vi "Main.vi"(11 "Module Admin":refnum<class "Delacor_lib_QMH_Cloneable Module Admin.lvclass">) -> ()   [LabVIEW 2025, in "Power Supply.lvlib"]
doc: "This template is based off of the Queued Message Handler design pattern and the Queued Message Handler project template that ships with LabVIEW.\n\nThe main difference is that the queue is private to this module and communication between modules is performed via Broadcast and Request events.\n\nRequest events are wrapped in public API methods and are handled in the Event Handling Loop (EHL) of this VI. Any module can register for Broadcast events sent by this module. The EHL generates messages based on user interface actions.\n\nThe Message Handling Loop (MHL) processes messages generated by the EHL, or by other messages. The messages are string values, so new messages can be added easily to the Message Cases case structure in the MHL. Each message cluster can also provide an optional value for Message Data, which is a variant that can be converted to whatever message-specific data is required.\n_____\nBased on DQMH Dev Tools: Project Template 7.1.2.1547."
uses:
  Power Supply.lvlib
  <vilib>/Delacor/Delacor QMH/Libraries/Message Queue_class/Delacor_lib_QMH_Message Queue.lvclass/Delacor_lib_QMH_Message Queue.ctl
  <vilib>/Delacor/Delacor QMH/Libraries/Cloneable Module Admin_class/Delacor_lib_QMH_Cloneable Module Admin.lvclass/Delacor_lib_QMH_Cloneable Module Admin.ctl
  <vilib>/Delacor/Delacor QMH/Libraries/Module Admin_class/Delacor_lib_QMH_Module Admin.lvclass/Delacor_lib_QMH_Module Admin.ctl
  <vilib>/Delacor/Delacor QMH/Libraries/Message Queue_class/Delacor_lib_QMH_Message Queue.lvclass
  Module Data--cluster.ctl
  <vilib>/Utility/miscctls.llb/LVPointTypeDef.ctl
  <vilib>/Delacor/Delacor QMH/Libraries/Message Queue_class/Delacor_lib_QMH_Enqueue Message (Single).vi
  Stop Argument--cluster.ctl
  <vilib>/Delacor/Delacor QMH/Libraries/Cloneable Module Admin_class/Delacor_lib_QMH_Cloneable Module Admin.lvclass
  select child (Reply Payload)--cluster.ctl
  Classes/hardware-selection.ctl
  select child Argument--cluster.ctl
  Classes/generic-power-supply/generic-power-supply.lvclass
  Classes/PSP-603/PSP-603.lvclass
  read config (Reply Payload)--cluster.ctl
  read config Argument--cluster.ctl
  init device (Reply Payload)--cluster.ctl
  init device Argument--cluster.ctl
  close (Reply Payload)--cluster.ctl
  close Argument--cluster.ctl
  output (Reply Payload)--cluster.ctl
  output Argument--cluster.ctl
  set voltage (Reply Payload)--cluster.ctl
  set voltage Argument--cluster.ctl
  set current (Reply Payload)--cluster.ctl
  set current Argument--cluster.ctl
  C:/Users/grove/Desktop/LabVIEW/Git/dqmh-lvoop-template/Libraries/Power Supply/Classes/generic-power-supply/generic-power-supply.lvclass
  C:/Users/grove/Desktop/LabVIEW/Git/dqmh-lvoop-template/Libraries/Power Supply/Classes/PSP-603/PSP-603.lvclass
panel:
  out "error out":errorcluster
  out "Status":string
  in  "Simulate EHL Error":bool
  in  "Simulate MHL Error":bool
  # "Other processes communicate with this Module via its Public API (wrappers for its Request Events).\n\nThis Module communicates with other processes via its Broadcast Events.\nAny process that wants to receive these messages can register for this module's Broadcast events."
  # "This template is for the DQMH framework. See the block diagram for more information on how to use this template."
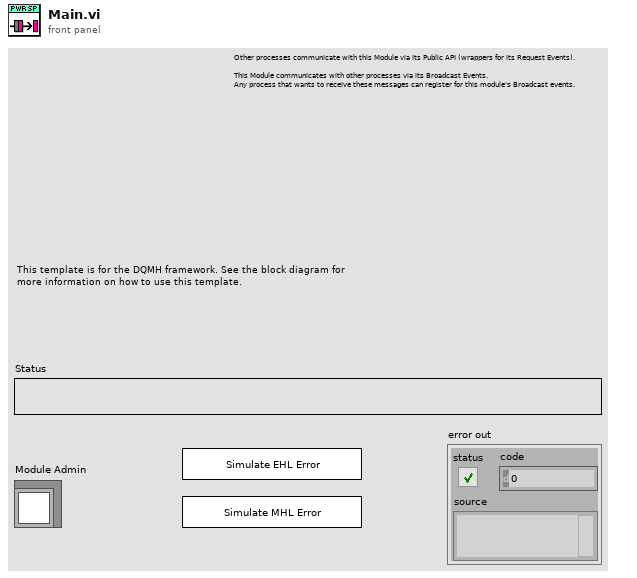
[diagram p1: front panel]
types:
  T1 = typedef "Power Supply.lvlib/Request Events--cluster.ctl" = cluster{"Stop Module":refnum<user-event>, "Show Panel":refnum<user-event>, "Hide Panel":refnum<user-event>, "Show Diagram":refnum<user-event>, "Get Module Execution Status":refnum<user-event>, "select child":refnum<user-event>, "read config":refnum<user-event>, "init device":refnum<user-event>, "close":refnum<user-event>, "output":refnum<user-event>, "set voltage":refnum<user-event>, "set current":refnum<user-event>}
  T2 = typedef "Power Supply.lvlib/Module Data--cluster.ctl" = cluster{"Status":string, "Power Supply Object":refnum<class "generic-power-supply.lvclass">}
  T3 = enum32{"invalid lock state", "Not Locked", "Locked (No Password)", "Password-protected"}
  T4 = typedef "Power Supply.lvlib/Stop Argument--cluster.ctl" = cluster{"Module ID":i32, "Origin":string, "Exit via Stop Module Req?":bool, "Wait for Module to stop?":bool}
  T5 = typedef "Power Supply.lvlib/select child Argument--cluster.ctl" = cluster{"Module ID":i32, "Enum":T6, "Wait Notifier":refnum<notifier>, "wait for reply":bool}
  T6 = typedef "hardware-selection.ctl" = enum16{"Parent", "Simulation", "PSP-603"}
  T7 = typedef "Power Supply.lvlib/read config Argument--cluster.ctl" = cluster{"Module ID":i32, "config json file":path, "Wait Notifier":refnum<notifier>, "wait for reply":bool}
  T8 = typedef "Power Supply.lvlib/init device Argument--cluster.ctl" = cluster{"Module ID":i32, "Variant":variant, "Wait Notifier":refnum<notifier>, "wait for reply":bool}
  T9 = typedef "Power Supply.lvlib/close Argument--cluster.ctl" = cluster{"Module ID":i32, "Wait Notifier":refnum<notifier>, "wait for reply":bool}
  T10 = typedef "Power Supply.lvlib/output Argument--cluster.ctl" = cluster{"Module ID":i32, "Output On/Off":bool, "Wait Notifier":refnum<notifier>, "wait for reply":bool}
  T11 = typedef "Power Supply.lvlib/set voltage Argument--cluster.ctl" = cluster{"Module ID":i32, "Output Voltage":dbl, "Wait Notifier":refnum<notifier>, "wait for reply":bool}
  T12 = typedef "Power Supply.lvlib/set current Argument--cluster.ctl" = cluster{"Module ID":i32, "Output Current":dbl, "Wait Notifier":refnum<notifier>, "wait for reply":bool}
  T13 = typedef "LVPointTypeDef.ctl" = cluster{"Horizontal":i16, "Vertical":i16}
  T14 = enum32{"Invalid", "Standard", "Closed", "Hidden", "Minimized", "Maximized"}
  T15 = typedef "Power Supply.lvlib/select child (Reply Payload)--cluster.ctl" = cluster{"Module ID":i32, "error":errorcluster}
  T16 = typedef "Power Supply.lvlib/read config (Reply Payload)--cluster.ctl" = cluster{"Module ID":i32, "error":errorcluster}
  T17 = typedef "Power Supply.lvlib/init device (Reply Payload)--cluster.ctl" = cluster{"Module ID":i32, "error":errorcluster}
  T18 = typedef "Power Supply.lvlib/close (Reply Payload)--cluster.ctl" = cluster{"Module ID":i32, "error":errorcluster}
  T19 = typedef "Power Supply.lvlib/output (Reply Payload)--cluster.ctl" = cluster{"Module ID":i32, "error":errorcluster}
  T20 = typedef "Power Supply.lvlib/set voltage (Reply Payload)--cluster.ctl" = cluster{"Module ID":i32, "error":errorcluster}
  T21 = typedef "Power Supply.lvlib/set current (Reply Payload)--cluster.ctl" = cluster{"Module ID":i32, "error":errorcluster}
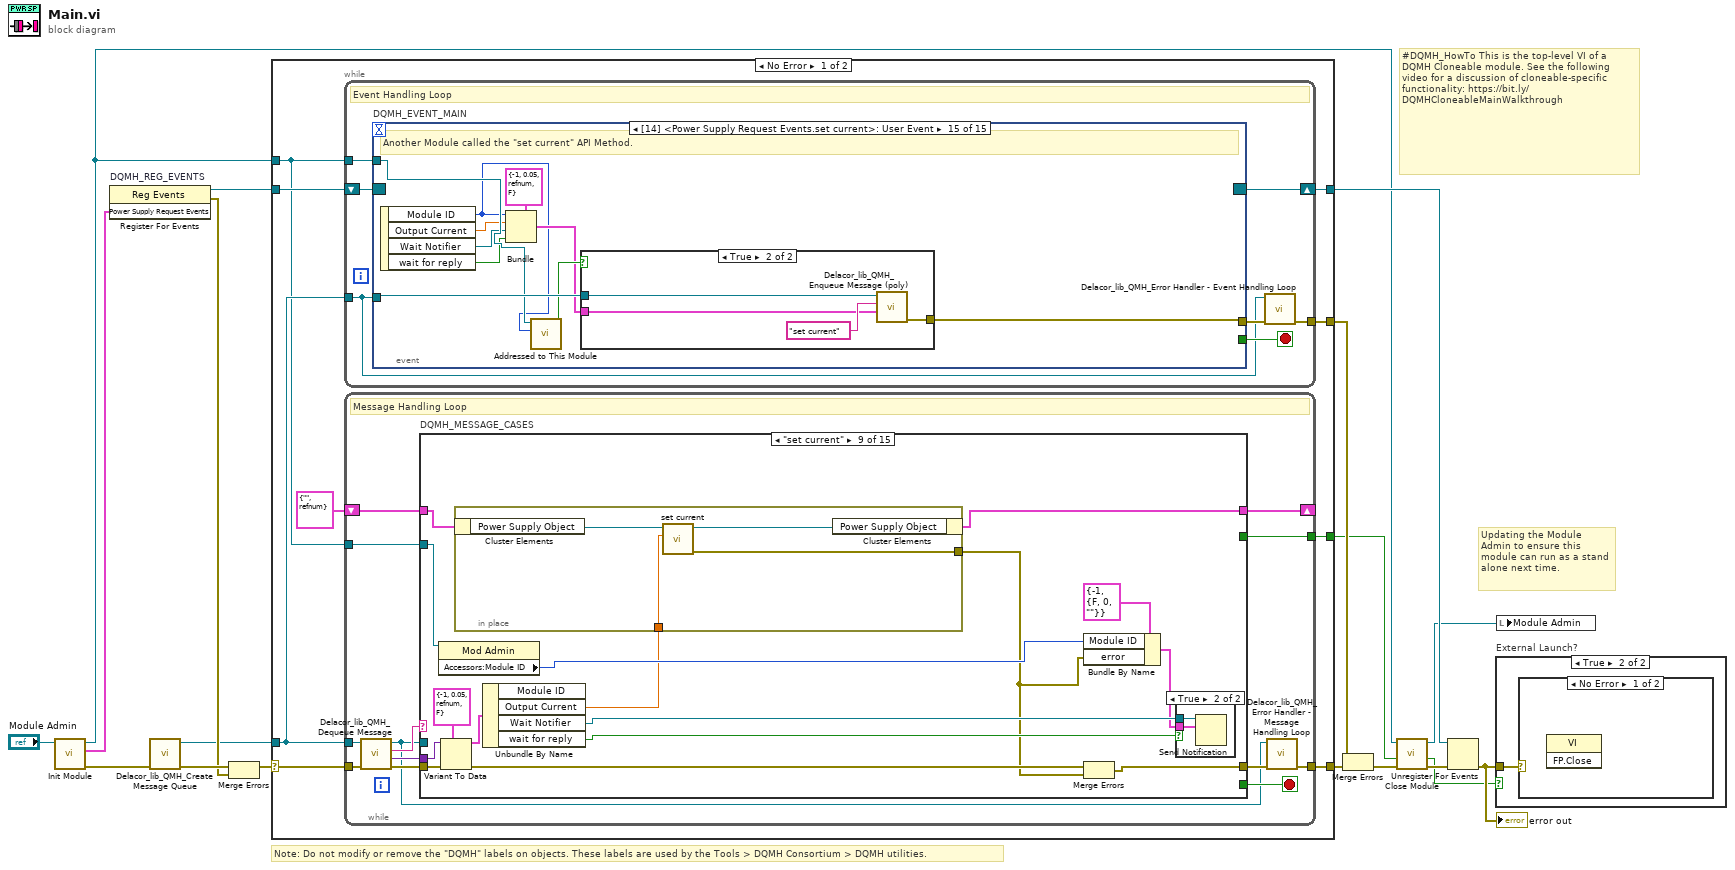
[diagram p0: block diagram]
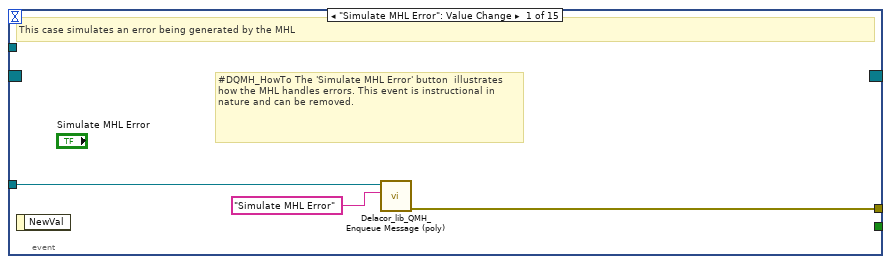
[diagram p2: hidden frame]
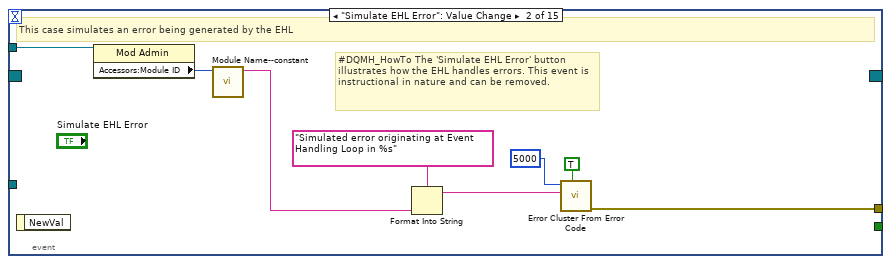
[diagram p3: hidden frame]
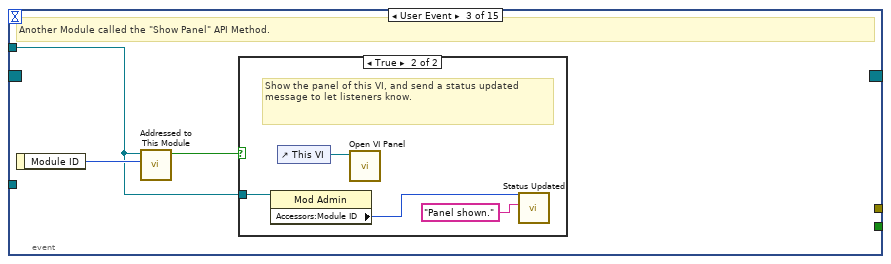
[diagram p4: hidden frame]
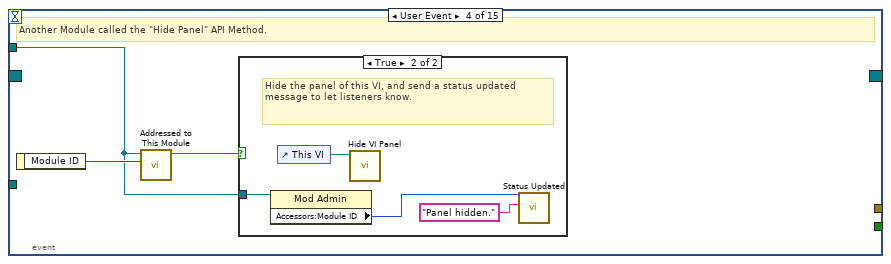
[diagram p6: hidden frame]
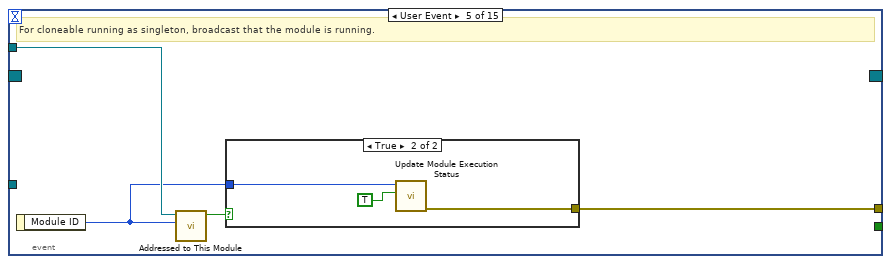
[diagram p8: hidden frame]
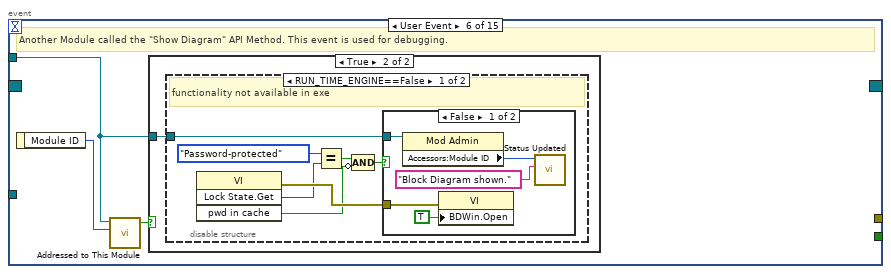
[diagram p10: hidden frame]
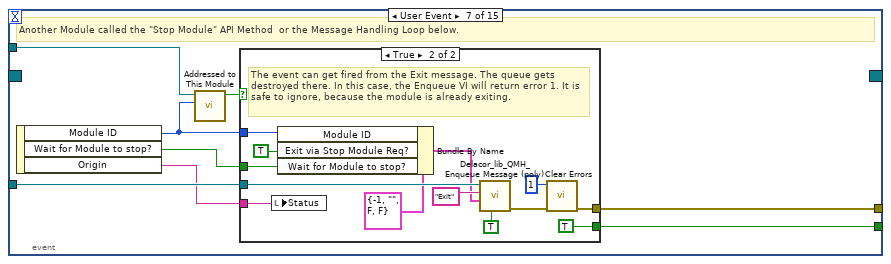
[diagram p14: hidden frame]
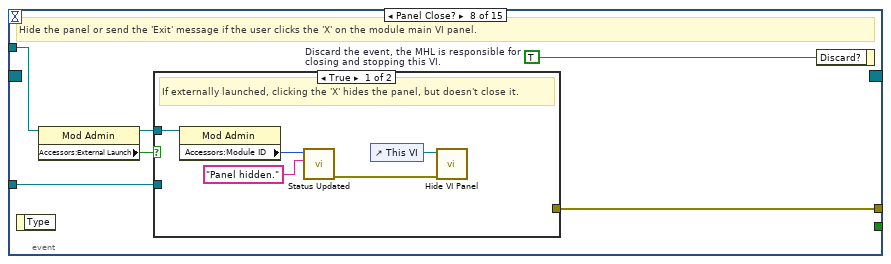
[diagram p16: hidden frame]
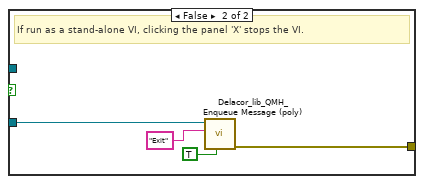
[diagram p17: hidden frame]
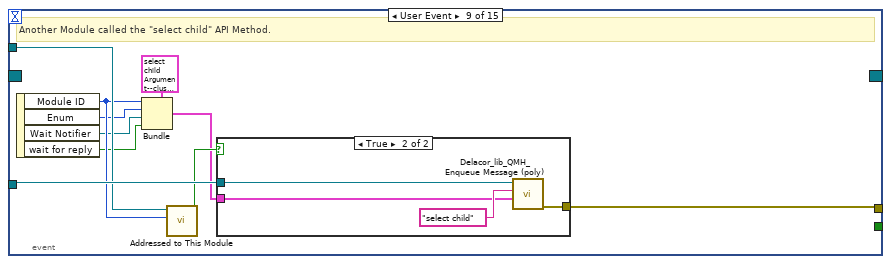
[diagram p18: hidden frame]
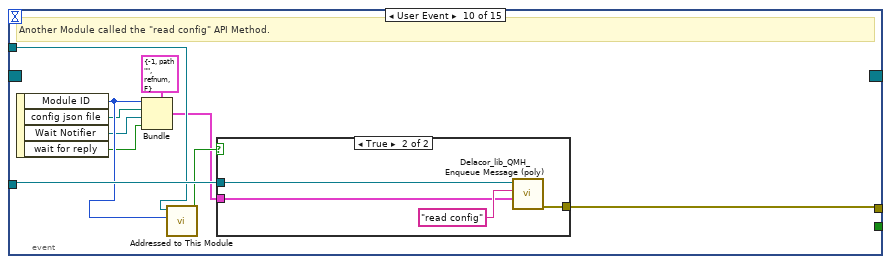
[diagram p20: hidden frame]
diagram:
  # "#DQMH_HowTo This is the top-level VI of a DQMH Cloneable module. See the following video for a discussion of cloneable-specific functionality: https://bit.ly/DQMHCloneableMainWalkthrough"
  # "Note: Do not modify or remove the \"DQMH\" labels on objects. These labels are used by the Tools > DQMH Consortium > DQMH utilities."
  # "Updating the Module Admin to ensure this module can run as a stand alone next time."
  n1 = call "Init Module.vi"("Cloneable Module Admin in"="Module Admin") -> ("error out"=w15:errorcluster, "Power Supply Request Events"=w7:T1, "Cloneable Module Admin out"=w4:refnum<class "Delacor_lib_QMH_Cloneable Module Admin.lvclass">)  [unwired: 8 in]
  n2 = register-events "DQMH_REG_EVENTS"(w7) -> (reference out=w8:refnum<event-registration>, error out=w10:errorcluster)  [unwired: 2 in]
  n3 = call <vilib>:"Delacor_lib_QMH_Create Message Queue.vi"("error in"=w15) -> ("error out"=w12:errorcluster, "Message Queue"=w6:refnum<class "Delacor_lib_QMH_Message Queue.lvclass">)  [unwired: 9 in]
  n4 = Merge Errors(w12, w10) -> (w11:errorcluster)
  n5 = case shown="No Error" w11 {
    selector: w11 -> [w25 w477]
    tunnel: [w27 w476] -> w16
    tunnel: [w24 w475] -> w9
    tunnel: w8 -> [w22 w475]
    tunnel: w6 -> [w21 w468]
    tunnel: [w26 _] -> w17
    tunnel: w4 -> [w20 w471]
    tunnel: [w19 _] -> w2
    frame No Error {
      n6 = while {
        tunnel: w21 -> [w28]
        shift-right: [w31] -> w24
        shift-left: w22 -> [w32]
        tunnel: [w33] -> w26
        tunnel: w20 -> [w29]
        stop <- w30 stop-if-true
        # "Event Handling Loop"
        n7 = event "DQMH_EVENT_MAIN" shown="[14] <Power Supply Request Events.set current>: User Event" {
          selector: w32 -> [_ _ _ _ _ _ _ _ _ _ _ _ _ _ _]
          dyn-events: [_ _ _ _ _ _ _ _ _ _ _ _ _ _ _] -> w31
          timeout: _ -> [_ _ _ _ _ _ _ _ _ _ _ _ _ _ _]
          tunnel: [_ _ _ _ _ _ w86 _ _ _ _ _ _ _ _] -> w30
          tunnel: w28 -> [w36 _ _ _ _ _ w89 w106 w128 w142 w156 w169 w183 w197 w211]
          tunnel: [w37 w45 _ _ w63 _ w90 w109 w119 w133 w147 w161 w174 w188 w202] -> w34
          tunnel: w29 -> [_ w44 w46 w53 w61 w67 w88 w107 w126 w140 w154 w167 w181 w195 w209]
          event "Simulate MHL Error": Value Change {
            # "#DQMH_HowTo The 'Simulate MHL Error' button  illustrates how the MHL handles errors. This event is instructional in nature and can be removed."
            # "This case simulates an error being generated by the MHL"
            n8 = event-data() -> ()  [unwired: 1 in, 1 out]
            n9 = call-poly <vilib>:"Delacor_lib_QMH_Enqueue Message (poly).vi"("Message"="Simulate MHL Error", "Message Queue in"=w36) -> ("error out"=w37:errorcluster)  [unwired: 8 in, 1 out]
          }
          event "Simulate EHL Error": Value Change {
            # "#DQMH_HowTo The 'Simulate EHL Error' button  illustrates how the EHL handles errors. This event is instructional in nature and can be removed."
            # "This case simulates an error being generated by the EHL"
            n10 = event-data() -> ()  [unwired: 1 in, 1 out]
            n11 = property on="Property Node" class="Mod Admin"(reference=w44) -> ("Accessors:Module ID"=w43:i32)  [unwired: 1 in, 2 out]
            n12 = call "Module Name--constant.vi"("Module ID"=w43) -> ("Module Name"=w38:string)  [unwired: 10 in]
            n13 = Format Into String(format string="Simulated error originating at Event Handling Loop in %s", w38) -> (resulting string=w41:string)  [unwired: 2 in, 1 out]
            n14 = call <vilib>:"Error Cluster From Error Code.vi"("show call chain? (False)"=TRUE, "error message (\"\")"=w41, "error code (0)"=5000) -> ("error out"=w45:errorcluster)  [unwired: 6 in]
          }
          event User Event {
            # "Another Module called the \"Show Panel\" API Method."
            n15 = event-data() -> ("Module ID"=w47:i32)  [unwired: 1 in]
            n16 = call "Addressed to This Module.vi"("Module ID from Argument"=w47, "Module Admin"=w46) -> ("Addressed to this instance?"=w48:bool)  [unwired: 8 in, 1 out]
            n17 = case shown="True" w48 {
              tunnel: w46 -> [_ w50]
              frame False {
              }
              frame True {
                # "Show the panel of this VI, and send a status updated message to let listeners know."
                n18 = property on="Property Node" class="Mod Admin"(reference=w50) -> ("Accessors:Module ID"=w49:i32)  [unwired: 1 in, 2 out]
                n19 = control-ref of="This VI"() -> (w52:refnum<vi>)
                n20 = call "Open VI Panel.vi"("VI"=w52) -> ()  [unwired: 10 in, 1 out]
                n21 = call "Status Updated.vi"("Status"="Panel shown." ("format string"), "Module ID"=w49) -> ()  [unwired: 9 in, 1 out]
              }
            }
          }
          event User Event {
            # "Another Module called the \"Hide Panel\" API Method."
            n22 = event-data() -> ("Module ID"=w54:i32)  [unwired: 1 in]
            n23 = call "Addressed to This Module.vi"("Module ID from Argument"=w54, "Module Admin"=w53) -> ("Addressed to this instance?"=w55:bool)  [unwired: 8 in, 1 out]
            n24 = case shown="True" w55 {
              tunnel: w53 -> [_ w57]
              frame False {
              }
              frame True {
                # "Hide the panel of this VI, and send a status updated message to let listeners know."
                n25 = property on="Property Node" class="Mod Admin"(reference=w57) -> ("Accessors:Module ID"=w56:i32)  [unwired: 1 in, 2 out]
                n26 = control-ref of="This VI"() -> (w59:refnum<vi>)
                n27 = call "Hide VI Panel.vi"("VI"=w59) -> ()  [unwired: 10 in, 1 out]
                n28 = call "Status Updated.vi"("Status"="Panel hidden." ("format string"), "Module ID"=w56) -> ()  [unwired: 9 in, 1 out]
              }
            }
          }
          event User Event {
            # "For cloneable running as singleton, broadcast that the module is running."
            n29 = event-data() -> ("Module ID"=w60:i32)  [unwired: 1 in]
            n30 = call "Addressed to This Module.vi"("Module ID from Argument"=w60, "Module Admin"=w61) -> ("Addressed to this instance?"=w62:bool)  [unwired: 8 in, 1 out]
            n31 = case shown="True" w62 {
              tunnel: [_ w66] -> w63
              tunnel: w60 -> [_ w65]
              frame False {
              }
              frame True {
                n32 = call "Update Module Execution Status.vi"("Running?"=TRUE, "Module ID"=w65) -> ("error out"=w66:errorcluster)  [unwired: 9 in]
              }
            }
          }
          event User Event {
            # "Another Module called the \"Show Diagram\" API Method. This event is used for debugging."
            n33 = event-data() -> ("Module ID"=w68:i32)  [unwired: 1 in]
            n34 = call "Addressed to This Module.vi"("Module ID from Argument"=w68, "Module Admin"=w67) -> ("Addressed to this instance?"=w69:bool)  [unwired: 8 in, 1 out]
            n35 = case shown="True" w69 {
              tunnel: w67 -> [_ w70]
              frame False {
              }
              frame True {
                n36 = disable-structure shown="RUN_TIME_ENGINE==False" {
                  disable-tunnel: w70 -> [w71 _]
                  frame condition #0 (active) {
                    # "functionality not available in exe"
                    n37 = invoke on="Invoke Node" class="VI" method="Lock State.Get"() -> (error out=w77:errorcluster, "Get Lock State"=w76:T3, "pwd in cache"=w73:bool)  [unwired: 4 in, 1 out]
                    n38 = Equal?(x=T3."Password-protected", y=w76) -> (x = y?=w74:bool)
                    n39 = Compound Arithmetic op=AND(w74, invert w73) -> (w72:bool)
                    n40 = case shown="False" w72 {
                      tunnel: w77 -> [w82 _]
                      tunnel: w71 -> [w79 _]
                      frame False {
                        n41 = property on="Property Node" class="Mod Admin"(reference=w79) -> ("Accessors:Module ID"=w78:i32)  [unwired: 1 in, 2 out]
                        n42 = property on="Property Node" class="VI"(error in=w82, "BDWin.Open"=TRUE ("Block Diagram Window:Open")) -> ()  [unwired: 1 in, 2 out]
                        n43 = call "Status Updated.vi"("Status"="Block Diagram shown." ("format string"), "Module ID"=w78) -> ()  [unwired: 9 in, 1 out]
                      }
                      frame True {
                        # "Password-protected VI, and the password is not in the cache. Do not show the diagram."
                      }
                    }
                  }
                  frame condition #1 {
                  }
                }
              }
            }
          }
          event User Event {
            # "Another Module called the \"Stop Module\" API Method  or the Message Handling Loop below."
            n44 = event-data() -> ("Module ID"=w84:i32, "Wait for Module to stop?"=w85:bool, "Origin"=w83:string)  [unwired: 1 in]
            n45 = call "Addressed to This Module.vi"("Module ID from Argument"=w84, "Module Admin"=w88) -> ("Addressed to this instance?"=w87:bool)  [unwired: 8 in, 1 out]
            n46 = case shown="True" w87 {
              tunnel: [_ w102] -> w90
              tunnel: w89 -> [_ w98]
              tunnel: [_ TRUE] -> w86
              tunnel: w85 -> [_ w93]
              tunnel: w84 -> [_ w95]
              tunnel: w83 -> [_ w91]
              frame False {
              }
              frame True {
                # "The event can get fired from the Exit message. The queue gets destroyed there. In this case, the Enqueue VI will return error 1. It is safe to ignore, because the module is already exiting."
                n47 = local write "Status"(w91) -> ()
                n48 = Bundle By Name(cluster=T4 {"Module ID"=-1, "Origin"="", "Exit via Stop Module Req?"=FALSE, "Wait for Module to stop?"=FALSE} ("Stop Argument"), "Module ID"=w95, "Exit via Stop Module Req?"=TRUE, "Wait for Module to stop?"=w93) -> (w92:T4)
                n49 = call-poly <vilib>:"Delacor_lib_QMH_Enqueue Message (poly).vi"("Priority Message? (F)"=TRUE, "Message Data"=w92, "Message"="Exit", "Message Queue in"=w98) -> ("error out"=w103:errorcluster)  [unwired: 6 in, 1 out]
                n50 = call <vilib>:"Clear Errors.vi"("error in (no error)"=w103, "specific error code to clear (0: all)"=1) -> ("error out"=w102:errorcluster)  [unwired: 4 in, 1 out]
              }
            }
          }
          event Panel Close? {
            w108 = TRUE  # Discard the event, the MHL is responsible for closing and stopping this VI.
            # "Hide the panel or send the 'Exit' message if the user clicks the 'X' on the module main VI panel."
            n51 = event-data() -> ()  [unwired: 1 in, 1 out]
            n52 = property on="Property Node" class="Mod Admin"(reference=w107) -> (reference out=w104:refnum<class "Delacor_lib_QMH_Cloneable Module Admin.lvclass">, "Accessors:External Launch"=w105:bool)  [unwired: 1 in, 1 out]
            n53 = case shown="True" w105 {
              tunnel: w106 -> [_ w117]
              tunnel: [_ w118] -> w109
              tunnel: w104 -> [w112 _]
              frame True {
                # "If externally launched, clicking the 'X' hides the panel, but doesn't close it."
                n54 = property on="Property Node" class="Mod Admin"(reference=w112) -> ("Accessors:Module ID"=w111:i32)  [unwired: 1 in, 2 out]
                n55 = call "Status Updated.vi"("Status"="Panel hidden." ("format string"), "Module ID"=w111) -> ("error out"=w110:errorcluster)  [unwired: 9 in]
                n56 = control-ref of="This VI"() -> (w114:refnum<vi>)
                n57 = call "Hide VI Panel.vi"("error in"=w110, "VI"=w114) -> ()  [unwired: 9 in, 1 out]
              }
              frame False {
                # "If run as a stand-alone VI, clicking the panel 'X' stops the VI."
                n58 = call-poly <vilib>:"Delacor_lib_QMH_Enqueue Message (poly).vi"("Priority Message? (F)"=TRUE, "Message"="Exit", "Message Queue in"=w117) -> ("error out"=w118:errorcluster)  [unwired: 7 in, 1 out]
              }
            }
            n59 = event-data ("Event Filter Node")("Discard?"=w108) -> ()  [unwired: 1 in, 1 out]
          }
          event User Event {
            # "Another Module called the \"select child\" API Method."
            n60 = event-data() -> ("Module ID"=w123:i32, "Enum"=w122:T6, "Wait Notifier"=w121:refnum<notifier>, "wait for reply"=w120:bool)  [unwired: 1 in]
            n61 = Bundle(cluster=T5 {"Module ID"=-1, "Enum"=enum."PSP-603", "Wait Notifier"=refnum, "wait for reply"=FALSE} ("select child Argument"), "Module ID"=w123, "Enum"=w122, "Wait Notifier"=w121, "wait for reply"=w120) -> (w124:T5)
            n62 = call "Addressed to This Module.vi"("Module ID from Argument"=w123, "Module Admin"=w126) -> ("Addressed to this instance?"=w127:bool)  [unwired: 8 in, 1 out]
            n63 = case shown="True" w127 {
              tunnel: w128 -> [_ w132]
              tunnel: w124 -> [_ w130]
              tunnel: [_ w129] -> w119
              frame False {
              }
              frame True {
                n64 = call-poly <vilib>:"Delacor_lib_QMH_Enqueue Message (poly).vi"("Message Data"=w130, "Message"="select child", "Message Queue in"=w132) -> ("error out"=w129:errorcluster)  [unwired: 7 in, 1 out]
              }
            }
          }
          event User Event {
            # "Another Module called the \"read config\" API Method."
            n65 = event-data() -> ("Module ID"=w137:i32, "config json file"=w136:path, "Wait Notifier"=w135:refnum<notifier>, "wait for reply"=w134:bool)  [unwired: 1 in]
            n66 = Bundle(cluster=T7 {"Module ID"=-1, "config json file"=path "", "Wait Notifier"=refnum, "wait for reply"=FALSE} ("read config Argument"), "Module ID"=w137, "config json file"=w136, "Wait Notifier"=w135, "wait for reply"=w134) -> (w138:T7)
            n67 = call "Addressed to This Module.vi"("Module ID from Argument"=w137, "Module Admin"=w140) -> ("Addressed to this instance?"=w141:bool)  [unwired: 8 in, 1 out]
            n68 = case shown="True" w141 {
              tunnel: w142 -> [_ w146]
              tunnel: w138 -> [_ w144]
              tunnel: [_ w143] -> w133
              frame False {
              }
              frame True {
                n69 = call-poly <vilib>:"Delacor_lib_QMH_Enqueue Message (poly).vi"("Message Data"=w144, "Message"="read config", "Message Queue in"=w146) -> ("error out"=w143:errorcluster)  [unwired: 7 in, 1 out]
              }
            }
          }
          event User Event {
            # "Another Module called the \"init device\" API Method."
            n70 = event-data() -> ("Module ID"=w151:i32, "Variant"=w150:variant, "Wait Notifier"=w149:refnum<notifier>, "wait for reply"=w148:bool)  [unwired: 1 in]
            n71 = Bundle(cluster=T8 {"Module ID"=-1, "Variant"=variant, "Wait Notifier"=refnum, "wait for reply"=FALSE} ("init device Argument"), "Module ID"=w151, "Variant"=w150, "Wait Notifier"=w149, "wait for reply"=w148) -> (w152:T8)
            n72 = call "Addressed to This Module.vi"("Module ID from Argument"=w151, "Module Admin"=w154) -> ("Addressed to this instance?"=w155:bool)  [unwired: 8 in, 1 out]
            n73 = case shown="True" w155 {
              tunnel: w156 -> [_ w160]
              tunnel: w152 -> [_ w158]
              tunnel: [_ w157] -> w147
              frame False {
              }
              frame True {
                n74 = call-poly <vilib>:"Delacor_lib_QMH_Enqueue Message (poly).vi"("Message Data"=w158, "Message"="init device", "Message Queue in"=w160) -> ("error out"=w157:errorcluster)  [unwired: 7 in, 1 out]
              }
            }
          }
          event User Event {
            # "Another Module called the \"close\" API Method."
            n75 = event-data() -> ("Module ID"=w164:i32, "Wait Notifier"=w163:refnum<notifier>, "wait for reply"=w162:bool)  [unwired: 1 in]
            n76 = Bundle(cluster=T9 {"Module ID"=-1, "Wait Notifier"=refnum, "wait for reply"=FALSE} ("close Argument"), "Module ID"=w164, "Wait Notifier"=w163, "wait for reply"=w162) -> (w165:T9)
            n77 = call "Addressed to This Module.vi"("Module ID from Argument"=w164, "Module Admin"=w167) -> ("Addressed to this instance?"=w168:bool)  [unwired: 8 in, 1 out]
            n78 = case shown="True" w168 {
              tunnel: w169 -> [_ w173]
              tunnel: w165 -> [_ w171]
              tunnel: [_ w170] -> w161
              frame False {
              }
              frame True {
                n79 = call-poly <vilib>:"Delacor_lib_QMH_Enqueue Message (poly).vi"("Message Data"=w171, "Message"="close", "Message Queue in"=w173) -> ("error out"=w170:errorcluster)  [unwired: 7 in, 1 out]
              }
            }
          }
          event User Event {
            # "Another Module called the \"output\" API Method."
            n80 = event-data() -> ("Module ID"=w178:i32, "Output On/Off"=w177:bool, "Wait Notifier"=w176:refnum<notifier>, "wait for reply"=w175:bool)  [unwired: 1 in]
            n81 = Bundle(cluster=T10 {"Module ID"=-1, "Output On/Off"=FALSE, "Wait Notifier"=refnum, "wait for reply"=FALSE} ("output Argument"), "Module ID"=w178, "Output On/Off"=w177, "Wait Notifier"=w176, "wait for reply"=w175) -> (w179:T10)
            n82 = call "Addressed to This Module.vi"("Module ID from Argument"=w178, "Module Admin"=w181) -> ("Addressed to this instance?"=w182:bool)  [unwired: 8 in, 1 out]
            n83 = case shown="True" w182 {
              tunnel: w183 -> [_ w187]
              tunnel: w179 -> [_ w185]
              tunnel: [_ w184] -> w174
              frame False {
              }
              frame True {
                n84 = call-poly <vilib>:"Delacor_lib_QMH_Enqueue Message (poly).vi"("Message Data"=w185, "Message"="output", "Message Queue in"=w187) -> ("error out"=w184:errorcluster)  [unwired: 7 in, 1 out]
              }
            }
          }
          event User Event {
            # "Another Module called the \"set voltage\" API Method."
            n85 = event-data() -> ("Module ID"=w192:i32, "Output Voltage"=w191:dbl, "Wait Notifier"=w190:refnum<notifier>, "wait for reply"=w189:bool)  [unwired: 1 in]
            n86 = Bundle(cluster=T11 {"Module ID"=-1, "Output Voltage"=10.0, "Wait Notifier"=refnum, "wait for reply"=FALSE} ("set voltage Argument"), "Module ID"=w192, "Output Voltage"=w191, "Wait Notifier"=w190, "wait for reply"=w189) -> (w193:T11)
            n87 = call "Addressed to This Module.vi"("Module ID from Argument"=w192, "Module Admin"=w195) -> ("Addressed to this instance?"=w196:bool)  [unwired: 8 in, 1 out]
            n88 = case shown="True" w196 {
              tunnel: w197 -> [_ w201]
              tunnel: w193 -> [_ w199]
              tunnel: [_ w198] -> w188
              frame False {
              }
              frame True {
                n89 = call-poly <vilib>:"Delacor_lib_QMH_Enqueue Message (poly).vi"("Message Data"=w199, "Message"="set voltage", "Message Queue in"=w201) -> ("error out"=w198:errorcluster)  [unwired: 7 in, 1 out]
              }
            }
          }
          event User Event {
            # "Another Module called the \"set current\" API Method."
            n90 = event-data() -> ("Module ID"=w206:i32, "Output Current"=w205:dbl, "Wait Notifier"=w204:refnum<notifier>, "wait for reply"=w203:bool)  [unwired: 1 in]
            n91 = Bundle(cluster=T12 {"Module ID"=-1, "Output Current"=0.05, "Wait Notifier"=refnum, "wait for reply"=FALSE} ("set current Argument"), "Module ID"=w206, "Output Current"=w205, "Wait Notifier"=w204, "wait for reply"=w203) -> (w207:T12)
            n92 = call "Addressed to This Module.vi"("Module ID from Argument"=w206, "Module Admin"=w209) -> ("Addressed to this instance?"=w210:bool)  [unwired: 8 in, 1 out]
            n93 = case shown="True" w210 {
              tunnel: w211 -> [_ w215]
              tunnel: w207 -> [_ w213]
              tunnel: [_ w212] -> w202
              frame False {
              }
              frame True {
                n94 = call-poly <vilib>:"Delacor_lib_QMH_Enqueue Message (poly).vi"("Message Data"=w213, "Message"="set current", "Message Queue in"=w215) -> ("error out"=w212:errorcluster)  [unwired: 7 in, 1 out]
              }
            }
          }
        }
        n95 = call-dynamic "Delacor_lib_QMH_Error Handler - Event Handling Loop.vi"("error in"=w34, "Message Queue in"=w28) -> ("dup error in"=w33:errorcluster)  [unwired: 8 in, 1 out]
      }
      n96 = while {
        tunnel: w21 -> [w216]
        shift-right: [w223] -> _
        shift-left: T2 {"Status"="", "Power Supply Object"=refnum} ("Data Cluster") -> [w224]
        tunnel: w25 -> [w227]
        tunnel: [w225] -> w27
        tunnel: w20 -> [w218]
        tunnel: [w217] -> w19
        stop <- w222 stop-if-true
        # "Message Handling Loop"
        n97 = call-dynamic "Delacor_lib_QMH_Dequeue Message.vi"("error in"=w227, "Message Queue in"=w216) -> ("error out"=w226:errorcluster, "Message Data"=w220:variant, "Message"=w221:string, "Message Queue out"=w219:refnum<class "Delacor_lib_QMH_Message Queue.lvclass">)  [unwired: 6 in]
        n98 = case "DQMH_MESSAGE_CASES" shown="\"set current\"" w221 {
          selector: w221 -> [_ _ _ _ _ _ _ _ _ _ _ _ _ _ w457]
          tunnel: w219 -> [_ _ _ _ _ _ _ _ _ _ _ w412 _ w449 _]
          tunnel: w226 -> [w247 w251 w267 w290 w312 w333 w354 w376 w398 w407 w409 w421 w438 w455 w466]
          tunnel: [w245 w251 w258 w281 w303 w324 w345 w367 w389 w406 w409 w417 w437 w450 w467] -> w228
          tunnel: w224 -> [w238 w250 w255 w278 w300 w321 w342 w364 w386 w405 w408 w416 w435 w448 w464]
          tunnel: [w237 w250 w254 w277 w299 w320 w341 w363 w385 w405 w408 w416 w435 w448 w464] -> w223
          tunnel: [_ _ _ _ _ _ _ _ _ _ _ _ _ w447 _] -> w222
          tunnel: w220 -> [_ _ w265 w288 w310 w331 w352 w374 w396 _ _ w415 _ w445 _]
          tunnel: w218 -> [w233 _ w256 w279 w301 w322 w343 w365 w387 _ _ w414 w433 w440 w463]
          tunnel: [_ _ _ _ _ _ _ _ _ _ _ _ _ w443 _] -> w217
          frame "Initialize" {
            w230 = "Initial Message" ("Initial Message")
            # "#DQMH_CodeNeeded - Initialize the appearance of the front panel."
            # "#DQMH_CodeNeeded - Initialize your state data here."
            # "Initialize - Any operation that needs to be done before the module can receive messages. Synchronize Caller Events.vi will inform Start Module.vi that the module has launched and is ready to receive messages. Module Did Init.vi will broadcast that the module initialized."
            n99 = call "Synchronize Caller Events.vi"("error in"=w247, "Module Admin"=w233) -> ("error out"=w246:errorcluster, "Module Admin out"=w232:refnum<class "Delacor_lib_QMH_Cloneable Module Admin.lvclass">)  [unwired: 8 in]
            n100 = property on="Property Node" class="Mod Admin"(reference=w232) -> ("Accessors:Module ID"=w229:i32, "Accessors:External Launch"=w234:bool)  [unwired: 1 in, 2 out]
            n101 = call "Module Name--constant.vi"("Module ID"=w229) -> ("Module Name"=w242:string)  [unwired: 10 in]
            n102 = property on="Property Node" class="VI"("Front Panel.Title"=w242) -> (reference out=w244:refnum<vi>, error out=w249:errorcluster)  [unwired: 2 in]
            n103 = Select(t=T14."Hidden" ("State"), s=w234, f=T14."Standard" ("State")) -> (s? t:f=w239:T14)
            n104 = invoke on="Invoke Node" class="VI" method="FP.Open"(reference=w244, error in=w249, "State"=w239) -> (reference out=w243:refnum<vi>, error out=w248:errorcluster)  [unwired: 2 in, 3 out]
            n105 = Bundle By Name(cluster=w238, "Status"=w230) -> (w237:T2)
            n106 = invoke on="Invoke Node" class="VI" method="FP.Center"(reference=w243, error in=w248) -> ()  [unwired: 1 in, 3 out]
            n107 = property on="Pane" class="Pane"("Origin"=T13 {"Horizontal"=0, "Vertical"=0}) -> ()  [unwired: 2 in, 2 out]
            n108 = call "Module Name--constant.vi"("Module ID"=w229) -> ("Module Name"=w235:string)  [unwired: 10 in]
            n109 = call "Module Did Init.vi"("error in"=w246, "Initialized?"=TRUE, "Origin"=w235, "Module ID"=w229) -> ("error out"=w245:errorcluster)  [unwired: 7 in]
            "Status" <- w230
          }
          frame "---Module Specific---" {
            # "Separator -- The following cases handle messages specific to this Module."
          }
          frame "select child" {
            w253 = errorcluster {"status"=FALSE, "code"=0, "source"=""} ("error")
            n110 = Variant To Data(error in=w267, type=T5 {"Module ID"=-1, "Enum"=enum."PSP-603", "Wait Notifier"=refnum, "wait for reply"=FALSE} ("select child Argument"), Variant=w265) -> (data=w263:T5, error out=w266:errorcluster)
            n111 = property class="Mod Admin"(reference=w256) -> ("Accessors:Module ID"=w257:i32)  [unwired: 1 in, 2 out]
            n112 = Unbundle By Name(w263) -> ("Enum"=w252:T6, "Wait Notifier"=w262:refnum<notifier>, "wait for reply"=w261:bool)  [unwired: 1 out]
            n113 = in-place {
              in-place-border: w252 -> [w268]
              n114 = in-place-cluster #1(w255) -> ()  [unwired: 1 out]
              n115 = case shown="\"Parent\"" w268 {
                tunnel: [refnum<class "generic-power-supply.lvclass"> refnum ("Power Supply.lvlib:generic-power-supply.lvclass") refnum<class "generic-power-supply.lvclass"> refnum ("Power Supply.lvlib:generic-power-supply.lvclass") refnum<class "PSP-603.lvclass"> refnum ("Power Supply.lvlib:PSP-603.lvclass")] -> w269
                frame "Simulation" {
                }
                frame "Parent" {
                }
                frame "PSP-603" {
                }
              }
              n116 = in-place-cluster #1("Power Supply Object"=w269) -> (w254:T2)
            }
            n117 = Bundle By Name(cluster=T15 {"Module ID"=-1, "error"={"status"=FALSE, "code"=0, "source"=""}} ("select child (Reply Payload)"), "Module ID"=w257, "error"=w253) -> (w260:T15)
            n118 = Merge Errors(w266, w253) -> (w258:errorcluster)
            n119 = case "DQMH_FIRE_NOTIFIER" shown="True" w261 {
              tunnel: w262 -> [_ w274]
              tunnel: w260 -> [_ w273]
              frame False {
              }
              frame True {
                n120 = Send Notification(notification=w273, notifier=w274) -> ()  [unwired: 1 in, 2 out]
              }
            }
          }
          frame "read config" {
            n121 = Variant To Data(error in=w290, type=T7 {"Module ID"=-1, "config json file"=path "", "Wait Notifier"=refnum, "wait for reply"=FALSE} ("read config Argument"), Variant=w288) -> (data=w286:T7, error out=w289:errorcluster)
            n122 = property class="Mod Admin"(reference=w279) -> ("Accessors:Module ID"=w280:i32)  [unwired: 1 in, 2 out]
            n123 = Unbundle By Name(w286) -> ("config json file"=w276:path, "Wait Notifier"=w285:refnum<notifier>, "wait for reply"=w284:bool)  [unwired: 1 out]
            n124 = in-place {
              in-place-border: w276 -> [w292]
              in-place-border: [w291] -> w275
              n125 = in-place-cluster #2(w278) -> ("Power Supply Object"=w294:refnum<class "generic-power-supply.lvclass">)
              n126 = call-dynamic "read config.vi"("File Path"=w292, "generic-power-supply in"=w294) -> ("error out"=w291:errorcluster, "generic-power-supply out"=w293:refnum<class "generic-power-supply.lvclass">)  [unwired: 8 in]
              n127 = in-place-cluster #2("Power Supply Object"=w293) -> (w277:T2)
            }
            n128 = Bundle By Name(cluster=T16 {"Module ID"=-1, "error"={"status"=FALSE, "code"=0, "source"=""}} ("read config (Reply Payload)"), "Module ID"=w280, "error"=w275) -> (w283:T16)
            n129 = Merge Errors(w289, w275) -> (w281:errorcluster)
            n130 = case "DQMH_FIRE_NOTIFIER" shown="True" w284 {
              tunnel: w285 -> [_ w296]
              tunnel: w283 -> [_ w295]
              frame False {
              }
              frame True {
                n131 = Send Notification(notification=w295, notifier=w296) -> ()  [unwired: 1 in, 2 out]
              }
            }
          }
          frame "init device" {
            n132 = Variant To Data(error in=w312, type=T8 {"Module ID"=-1, "Variant"=variant, "Wait Notifier"=refnum, "wait for reply"=FALSE} ("init device Argument"), Variant=w310) -> (data=w308:T8, error out=w311:errorcluster)
            n133 = property class="Mod Admin"(reference=w301) -> ("Accessors:Module ID"=w302:i32)  [unwired: 1 in, 2 out]
            n134 = Unbundle By Name(w308) -> ("Variant"=w297:variant, "Wait Notifier"=w307:refnum<notifier>, "wait for reply"=w306:bool)  [unwired: 1 out]
            n135 = in-place {
              in-place-border: [w314] -> w298
              in-place-border: w297 -> [w313]
              n136 = in-place-cluster #3(w300) -> ("Power Supply Object"=w315:refnum<class "generic-power-supply.lvclass">)
              n137 = call-dynamic "init.vi"("Variant"=w313, "generic-power-supply in"=w315) -> ("error out"=w314:errorcluster, "generic-power-supply out"=w316:refnum<class "generic-power-supply.lvclass">)  [unwired: 8 in]
              n138 = in-place-cluster #3("Power Supply Object"=w316) -> (w299:T2)
            }
            n139 = Bundle By Name(cluster=T17 {"Module ID"=-1, "error"={"status"=FALSE, "code"=0, "source"=""}} ("init device (Reply Payload)"), "Module ID"=w302, "error"=w298) -> (w305:T17)
            n140 = Merge Errors(w311, w298) -> (w303:errorcluster)
            n141 = case "DQMH_FIRE_NOTIFIER" shown="True" w306 {
              tunnel: w307 -> [_ w318]
              tunnel: w305 -> [_ w317]
              frame False {
              }
              frame True {
                n142 = Send Notification(notification=w317, notifier=w318) -> ()  [unwired: 1 in, 2 out]
              }
            }
          }
          frame "close" {
            n143 = Variant To Data(error in=w333, type=T9 {"Module ID"=-1, "Wait Notifier"=refnum, "wait for reply"=FALSE} ("close Argument"), Variant=w331) -> (data=w329:T9, error out=w332:errorcluster)
            n144 = in-place {
              in-place-border: [w334] -> w319
              n145 = in-place-cluster #4(w321) -> ("Power Supply Object"=w336:refnum<class "generic-power-supply.lvclass">)
              n146 = call-dynamic "close.vi"("generic-power-supply in"=w336) -> ("error out"=w334:errorcluster, "generic-power-supply out"=w335:refnum<class "generic-power-supply.lvclass">)  [unwired: 9 in]
              n147 = in-place-cluster #4("Power Supply Object"=w335) -> (w320:T2)
            }
            n148 = property class="Mod Admin"(reference=w322) -> ("Accessors:Module ID"=w323:i32)  [unwired: 1 in, 2 out]
            n149 = Unbundle By Name(w329) -> ("Wait Notifier"=w328:refnum<notifier>, "wait for reply"=w327:bool)  [unwired: 1 out]
            n150 = Bundle By Name(cluster=T18 {"Module ID"=-1, "error"={"status"=FALSE, "code"=0, "source"=""}} ("close (Reply Payload)"), "Module ID"=w323, "error"=w319) -> (w326:T18)
            n151 = Merge Errors(w332, w319) -> (w324:errorcluster)
            n152 = case "DQMH_FIRE_NOTIFIER" shown="True" w327 {
              tunnel: w328 -> [_ w338]
              tunnel: w326 -> [_ w337]
              frame False {
              }
              frame True {
                n153 = Send Notification(notification=w337, notifier=w338) -> ()  [unwired: 1 in, 2 out]
              }
            }
          }
          frame "output" {
            n154 = property class="Mod Admin"(reference=w343) -> ("Accessors:Module ID"=w344:i32)  [unwired: 1 in, 2 out]
            n155 = Variant To Data(error in=w354, type=T10 {"Module ID"=-1, "Output On/Off"=FALSE, "Wait Notifier"=refnum, "wait for reply"=FALSE} ("output Argument"), Variant=w352) -> (data=w350:T10, error out=w353:errorcluster)
            n156 = Unbundle By Name(w350) -> ("Output On/Off"=w340:bool, "Wait Notifier"=w349:refnum<notifier>, "wait for reply"=w348:bool)  [unwired: 1 out]
            n157 = in-place {
              in-place-border: w340 -> [w356]
              in-place-border: [w355] -> w339
              n158 = in-place-cluster #5(w342) -> ("Power Supply Object"=w358:refnum<class "generic-power-supply.lvclass">)
              n159 = call-dynamic "output.vi"("Output [on/off]"=w356, "generic-power-supply in"=w358) -> ("error out"=w355:errorcluster, "generic-power-supply out"=w357:refnum<class "generic-power-supply.lvclass">)  [unwired: 8 in]
              n160 = in-place-cluster #5("Power Supply Object"=w357) -> (w341:T2)
            }
            n161 = Bundle By Name(cluster=T19 {"Module ID"=-1, "error"={"status"=FALSE, "code"=0, "source"=""}} ("output (Reply Payload)"), "Module ID"=w344, "error"=w339) -> (w347:T19)
            n162 = Merge Errors(w353, w339) -> (w345:errorcluster)
            n163 = case "DQMH_FIRE_NOTIFIER" shown="True" w348 {
              tunnel: w349 -> [_ w360]
              tunnel: w347 -> [_ w359]
              frame False {
              }
              frame True {
                n164 = Send Notification(notification=w359, notifier=w360) -> ()  [unwired: 1 in, 2 out]
              }
            }
          }
          frame "set voltage" {
            n165 = Variant To Data(error in=w376, type=T11 {"Module ID"=-1, "Output Voltage"=10.0, "Wait Notifier"=refnum, "wait for reply"=FALSE} ("set voltage Argument"), Variant=w374) -> (data=w372:T11, error out=w375:errorcluster)
            n166 = property class="Mod Admin"(reference=w365) -> ("Accessors:Module ID"=w366:i32)  [unwired: 1 in, 2 out]
            n167 = Unbundle By Name(w372) -> ("Output Voltage"=w362:dbl, "Wait Notifier"=w371:refnum<notifier>, "wait for reply"=w370:bool)  [unwired: 1 out]
            n168 = in-place {
              in-place-border: w362 -> [w378]
              in-place-border: [w377] -> w361
              n169 = in-place-cluster #6(w364) -> ("Power Supply Object"=w380:refnum<class "generic-power-supply.lvclass">)
              n170 = call-dynamic "set voltage.vi"("Voltage"=w378, "generic-power-supply in"=w380) -> ("error out"=w377:errorcluster, "generic-power-supply out"=w379:refnum<class "generic-power-supply.lvclass">)  [unwired: 8 in]
              n171 = in-place-cluster #6("Power Supply Object"=w379) -> (w363:T2)
            }
            n172 = Bundle By Name(cluster=T20 {"Module ID"=-1, "error"={"status"=FALSE, "code"=0, "source"=""}} ("set voltage (Reply Payload)"), "Module ID"=w366, "error"=w361) -> (w369:T20)
            n173 = Merge Errors(w375, w361) -> (w367:errorcluster)
            n174 = case "DQMH_FIRE_NOTIFIER" shown="True" w370 {
              tunnel: w371 -> [_ w382]
              tunnel: w369 -> [_ w381]
              frame False {
              }
              frame True {
                n175 = Send Notification(notification=w381, notifier=w382) -> ()  [unwired: 1 in, 2 out]
              }
            }
          }
          frame "set current" {
            n176 = property class="Mod Admin"(reference=w387) -> ("Accessors:Module ID"=w388:i32)  [unwired: 1 in, 2 out]
            n177 = Variant To Data(error in=w398, type=T12 {"Module ID"=-1, "Output Current"=0.05, "Wait Notifier"=refnum, "wait for reply"=FALSE} ("set current Argument"), Variant=w396) -> (data=w394:T12, error out=w397:errorcluster)
            n178 = Unbundle By Name(w394) -> ("Output Current"=w384:dbl, "Wait Notifier"=w393:refnum<notifier>, "wait for reply"=w392:bool)  [unwired: 1 out]
            n179 = in-place {
              in-place-border: w384 -> [w400]
              in-place-border: [w399] -> w383
              n180 = in-place-cluster #7(w386) -> ("Power Supply Object"=w402:refnum<class "generic-power-supply.lvclass">)
              n181 = call-dynamic "set current.vi"("Current [A]"=w400, "generic-power-supply in"=w402) -> ("error out"=w399:errorcluster, "generic-power-supply out"=w401:refnum<class "generic-power-supply.lvclass">)  [unwired: 8 in]
              n182 = in-place-cluster #7("Power Supply Object"=w401) -> (w385:T2)
            }
            n183 = Bundle By Name(cluster=T21 {"Module ID"=-1, "error"={"status"=FALSE, "code"=0, "source"=""}} ("set current (Reply Payload)"), "Module ID"=w388, "error"=w383) -> (w391:T21)
            n184 = Merge Errors(w397, w383) -> (w389:errorcluster)
            n185 = case "DQMH_FIRE_NOTIFIER" shown="True" w392 {
              tunnel: w393 -> [_ w404]
              tunnel: w391 -> [_ w403]
              frame False {
              }
              frame True {
                n186 = Send Notification(notification=w403, notifier=w404) -> ()  [unwired: 1 in, 2 out]
              }
            }
          }
          frame "---Copy This Frame---" {
            # "Duplicate this frame when creating new messages.  Change this comment in the duplicated frame to describe this message."
            n187 = Merge Errors(w407) -> (w406:errorcluster)
          }
          frame "---Exit and Error Handling---" {
            # "Separator - the following cases handle errors and exit messages."
          }
          frame "Error" {
            # "#DQMH_CodeRecommended - If the module is running in standalone mode (External Launch = FALSE), this code will pop up an error dialog and call the 'Exit' message if an error occurs. Add more fine-grained error management here."
            # "Error - Check the error message data and respond accordingly. This message is sent by the \"Error Handler\" VIs at the end of each loop in this application."
            n188 = property on="Property Node" class="Mod Admin"(reference=w414) -> ("Accessors:External Launch"=w413:bool, "Accessors:Module ID"=w411:i32)  [unwired: 1 in, 2 out]
            n189 = Variant To Data(error in=w421, type=errorcluster {"status"=FALSE, "code"=0, "source"=""} ("error constant"), Variant=w415) -> (data=w410:errorcluster, error out=w419:errorcluster)
            n190 = local write "error out"(w410) -> ()
            n191 = call "Error Reported.vi"("Error"=w410, "Module ID"=w411) -> ()  [unwired: 9 in, 1 out]
            n192 = case shown="False" w413 {
              tunnel: [w426 _] -> w418
              tunnel: w412 -> [w424 _]
              tunnel: w410 -> [w425 _]
              frame False {
                n193 = disable-structure shown="Default" {
                  disable-tunnel: w425 -> [w427 _]
                  frame condition #0 (active) {
                    # "If the module is running standalone, then pop up an error dialog and call the \"Exit\" message."
                    n194 = call <vilib>:"Simple Error Handler.vi"("error in (no error)"=w427) -> ()  [unwired: 4 in, 5 out]
                  }
                  frame condition #1 {
                    # "To prevent the Simple Error Handler VI from being loaded (e.g. when deploying to a Real-Time target), add the Conditional Disable Symbol \"DQMH_Disable_SEH\" to your project and set it to TRUE."
                  }
                }
                n195 = call-poly <vilib>:"Delacor_lib_QMH_Enqueue Message (poly).vi"("Priority Message? (F)"=TRUE, "Message"="Exit", "Message Queue in"=w424) -> ("error out"=w426:errorcluster)  [unwired: 7 in, 1 out]
              }
              frame True {
                # "If the module was launched externally, calling the Error Reported broadcast VI is the only action performed by the \"Error\" message. The module's caller can then process the error appropriately."
              }
            }
            n196 = Merge Errors(w419, w418) -> (w417:errorcluster)
          }
          frame "Simulate MHL Error" {
            # "#DQMH_HowTo The 'Simulate MHL Error' button  illustrates how the MHL handles errors. This event is instructional in nature and can be removed."
            # "Simulate an error occurring at the MHL"
            n197 = property on="Property Node" class="Mod Admin"(reference=w433) -> ("Accessors:Module ID"=w434:i32)  [unwired: 1 in, 2 out]
            n198 = call "Module Name--constant.vi"("Module ID"=w434) -> ("Module Name"=w429:string)  [unwired: 10 in]
            n199 = Format Into String(format string="Simulated error originating at Message Handling Loop in %s", w429) -> (resulting string=w430:string)  [unwired: 2 in, 1 out]
            n200 = call <vilib>:"Error Cluster From Error Code.vi"("show call chain? (False)"=TRUE, "error message (\"\")"=w430, "error code (0)"=5001) -> ("error out"=w436:errorcluster)  [unwired: 6 in]
            n201 = Merge Errors(w438, w436) -> (w437:errorcluster)
          }
          frame "Exit" {
            w446 = 91  # 91: not all Exit messages will have an argument
            w447 = TRUE  # Stop the VI
            # "Release the message queue reference"
            # "#DQMH_CodeNeeded - Add any required cleanup code here."
            # "Exit - Exit the application."
            n202 = Variant To Data(error in=w455, type=T4 {"Module ID"=-1, "Origin"="", "Exit via Stop Module Req?"=FALSE, "Wait for Module to stop?"=FALSE} ("Stop Argument"), Variant=w445) -> (data=w442:T4, error out=w451:errorcluster)
            n203 = call <vilib>:"Clear Errors.vi"("error in (no error)"=w451, "specific error code to clear (0: all)"=w446) -> ("error out"=w454:errorcluster)  [unwired: 4 in, 1 out]
            n204 = property on="Property Node" class="Mod Admin"(reference=w440) -> ("Accessors:Module ID"=w439:i32)  [unwired: 1 in, 2 out]
            n205 = control-ref of="This VI"() -> (w441:refnum<vi>)
            n206 = call-dynamic "Delacor_lib_QMH_Release Message Queue.vi"("error in"=w454, "Message Queue"=w449) -> ("error out"=w453:errorcluster)  [unwired: 9 in]
            n207 = call "Handle Exit.vi"("Stop Argument"=w442, "Module Admin in"=w440, "VI reference"=w441) -> ("error out"=w452:errorcluster, "Wait for Stop?"=w443:bool)  [unwired: 7 in]
            n208 = Merge Errors(w453, w452) -> (w450:errorcluster)
            n209 = call "Error Reported.vi"("Error"=w450, "Module ID"=w439) -> ()  [unwired: 9 in, 1 out]
          }
          frame Default {
            # "'Default' case only runs if there is a message that isn't defined in any of the other cases.  Output a programming error."
            n210 = property on="Property Node" class="Mod Admin"(reference=w463) -> ("Accessors:Module ID"=w462:i32)  [unwired: 1 in, 2 out]
            n211 = call "Module Name--constant.vi"("Module ID"=w462) -> ("Module Name"=w456:string)  [unwired: 10 in]
            n212 = Format Into String(format string="The invalid message string \"%s\" was received in the Message Handling Loop for module \"%s\".", w457, w456) -> (resulting string=w459:string)  [unwired: 2 in, 1 out]
            n213 = call <vilib>:"Error Cluster From Error Code.vi"("show call chain? (False)"=TRUE, "error message (\"\")"=w459, "error code (0)"=1) -> ("error out"=w465:errorcluster)  [unwired: 6 in]
            n214 = Merge Errors(w466, w465) -> (w467:errorcluster)
          }
        }
        n215 = call-dynamic "Delacor_lib_QMH_Error Handler - Message Handling Loop.vi"("error in"=w228, "Message Queue in"=w219) -> ("dup error in"=w225:errorcluster)  [unwired: 8 in, 1 out]
      }
    }
    frame Error {
      n216 = call "Synchronize Caller Events.vi"("Module Admin"=w471) -> ("Module Admin out"=w470:refnum<class "Delacor_lib_QMH_Cloneable Module Admin.lvclass">)  [unwired: 9 in, 1 out]
      n217 = property on="Property Node" class="Mod Admin"(reference=w470) -> ("Accessors:Module ID"=w469:i32)  [unwired: 1 in, 2 out]
      n218 = call-dynamic "Delacor_lib_QMH_Release Message Queue.vi"("error in"=w477, "Message Queue"=w468) -> ("error out"=w476:errorcluster)  [unwired: 9 in]
      n219 = call "Module Name--constant.vi"("Module ID"=w469) -> ("Module Name"=w474:string)  [unwired: 10 in]
      n220 = Format Into String(format string="An error occurred during initialization. %s is no longer running.", w474) -> (resulting string=w472:string)  [unwired: 2 in, 1 out]
      n221 = call "Error Reported.vi"("Additional Information"=w472, "Error"=w476, "Module ID"=w469) -> ()  [unwired: 8 in, 1 out]
    }
  }
  n222 = Merge Errors(w17, w16) -> (w18:errorcluster)
  n223 = call "Close Module.vi"("error in"=w18, "Wait for stop?"=w2, "Module Admin in"=w4) -> ("error out"=w14:errorcluster, "External Launch"=w1:bool, "Module Admin out"=w3:refnum<class "Delacor_lib_QMH_Cloneable Module Admin.lvclass">)  [unwired: 6 in]
  n224 = Unregister For Events(event registration refnum=w9, error in=w14) -> (error out=w13:errorcluster)
  "error out" <- w13
  n225 = case "External Launch?" shown="True" w1 {
    tunnel: w13 -> [_ w478]
    frame False {
    }
    frame True {
      n226 = case shown="No Error" w478 {
        frame No Error {
          n227 = invoke class="VI" method="FP.Close"() -> ()  [unwired: 3 in, 3 out]
        }
        frame Error {
          n228 = disable-structure shown="Default" {
            frame condition #0 (active) {
              n229 = invoke class="VI" method="FP.Open"("Activate"=TRUE ("Activate?")) -> ()  [unwired: 4 in, 5 out]
            }
            frame condition #1 {
              # "Don't show panel on error if running inside a built EXE."
            }
          }
        }
      }
    }
  }
  n230 = local write "Module Admin"(w3) -> ()
